vi "Semaphore Timed Wait.vi"(8 "error in (no error)":errorcluster, 10 "absolute timeout":T1, 11 "Semaphore in":T2) -> (0 "error out":errorcluster, 2 "timed out?":bool, 3 "Semaphore out":T2)   [LabVIEW 2013, in "POSIX Threads.lvlib" / "Semaphore.lvclass"]
doc: "Calls sem_timedwait() on a semaphore referenced by the provided Semaphore object. This function will wait for a sempahore with a value of 0 to be incremented to 1, and then subsequently decremenet the semaphore back to 0 before returning. If the semaphore value is not incremented to 1 before the specified timeout is reached, this function returns a timeout status of TRUE."
uses:
  Semaphore.lvclass
  Controls/reference.ctl
  <vilib>/NI/NI Linux RT Utilities/Controls/Public/C Structs/timespec_64.ctl
  POSIX Thread Object/POSIX Thread Object.lvclass/POSIX Thread Object.ctl
  POSIX Thread Object/Private VIs/libpthread path.vi
  <vilib>/NI/NI Linux RT Utilities/VIs/Public/Convert Types/convert timespec 64 to timespec 32.vi
  POSIX Thread Object/Private VIs/get pthread error.vi
  <vilib>/NI/NI Linux RT Errno/VIs/Public/Get Errno Value for Calling Thread.vi
  POSIX Thread Object/POSIX Thread Object.lvclass
  <vilib>/NI/NI Linux RT Utilities/Linux RT Utilities.lvlib
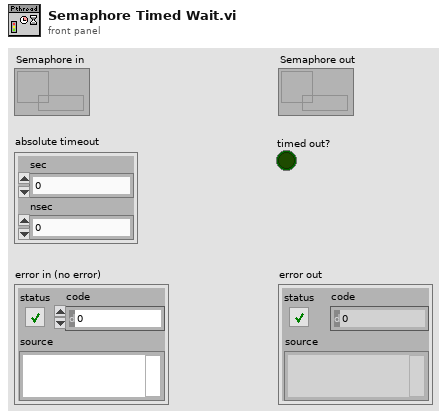
[diagram p1: front panel]
types:
  T1 = typedef "Linux RT Utilities.lvlib/timespec_64.ctl" = cluster{"sec":u64, "nsec":u64}
  T2 = typedef "POSIX Threads.lvlib/Semaphore.lvclass/reference.ctl" = refnum<data-value>
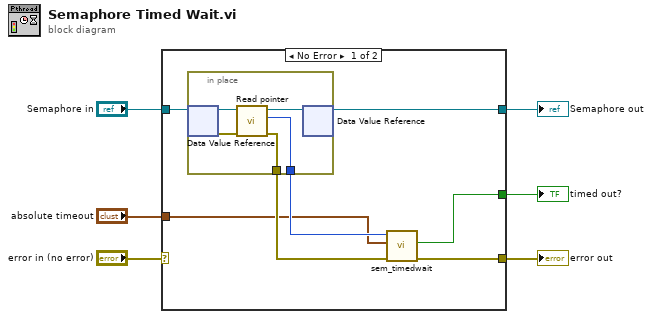
[diagram p0: block diagram]
diagram:
  n1 = case shown="No Error" "error in (no error)" {
    selector: "error in (no error)" -> [_ w19]
    tunnel: "Semaphore in" -> [w13 w20]
    tunnel: [w12 w20] -> w3
    tunnel: [w10 w19] -> w4
    tunnel: "absolute timeout" -> [w8 _]
    tunnel: [w7 _] -> w1
    frame No Error {
      n2 = in-place {
        in-place-border: [w15] -> w11
        in-place-border: [w14] -> w9
        n3 = in-place-dvr #1(w13) -> (w18:refnum<class "Semaphore.lvclass">, w17:errorcluster)
        n4 = call "Read pointer.vi"("error in (no error)"=w17, "POSIX Thread Object in"=w18) -> ("error out"=w15:errorcluster, "pointer"=w14:u64, "POSIX Thread Object out"=w16:refnum<class "Semaphore.lvclass">)  [unwired: 7 in]
        n5 = in-place-dvr #1(w16) -> (w12:T2)  [unwired: 1 out]
      }
      n6 = call "sem_timedwait.vi"("error in (no error)"=w11, "absolute timeout"=w8, "sempahore ptr in"=w9) -> ("error out"=w10:errorcluster, "timed out?"=w7:bool)  [unwired: 6 in, 1 out]
    }
    frame Error {
    }
  }
  "error out" <- w4
  "Semaphore out" <- w3
  "timed out?" <- w1
